vi "Begin_Tipper.vi"() -> (0 "error out":errorcluster)   [LabVIEW 2012]
uses:
  <vilib>/Rock Robotics/WPI/CAN/Jaguar/SubVIs/WPI_CANJaguar_BrakeCoastMode.ctl
  <vilib>/Rock Robotics/WPI/MotorControl/WPI_MotorControlOpenCANJaguar.vi
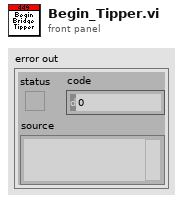
[diagram p1: front panel]
types:
  T1 = typedef "WPI_CANJaguar_BrakeCoastMode.ctl" = enum8{"Jumper", "Brake", "Coast"}
  T2 = typedef "WPI_MotorControlDeviceRef.ctl" = cluster{"DeviceStatus":errorcluster, "Type":enum16{"PWM", "CAN"}, "PWM":cluster{"Digital Module":T3, "PWM Channel":T4, "DeadBand":T5}, "CAN":cluster{"Device Number":u8, "Control Mode":T6, "Semaphore":T7, "Max Vout":dbl}, "Invert":bool, "TransformRef":T8, "InvTransformRef":T8}
  T3 = typedef "FPGA_TypedefDigitalModule.ctl" = enum16{"Digital Module 1", "Digital Module 2"}
  T4 = typedef "FPGA_DIOPWMChannel.ctl" = enum8{"PWM 1", "PWM 2", "PWM 3", "PWM 4", "PWM 5", "PWM 6", "PWM 7", "PWM 8", "PWM 9", "PWM 10", "Invalid"}
  T5 = typedef "WPI_PWMDeadband.ctl" = cluster{"Name":string, "maxPositivePwm":i32, "minPositivePwm":i32, "centerPwm":i32, "maxNegativePwm":i32, "minNegativePwm":i32, "angularRange":u16}
  T6 = typedef "WPI_CANJaguar_ControlMode.ctl" = enum8{"Percent VBus", "Current", "Speed", "Position", "Voltage"}
  T7 = typedef "Semaphore RefNum" = refnum<k1>
  T8 = typedef "WPI_PWMTransform_ConPane.ctl" = refnum<vi>
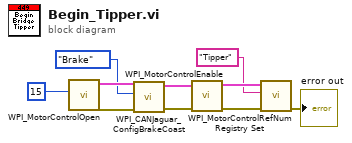
[diagram p0: block diagram]
diagram:
  n1 = call-poly <vilib>:"WPI_MotorControlOpen.vi"("Device Number"=u8 15) -> ("error out"=w3:errorcluster, "MotorControlDeviceRef"=w2:T2)  [unwired: 9 in]
  n2 = call <vilib>:"WPI_CANJaguar_ConfigBrakeCoast.vi"("error in (no error)"=w3, "Brake / Coast Mode"=WPI_CANJaguar_BrakeCoastMode."Brake", "CAN Jaguar Ref"=w2) -> ("error out"=w4:errorcluster, "CAN Jaguar Ref Out"=w5:T2)  [unwired: 7 in]
  n3 = call <vilib>:"WPI_MotorControlEnable.vi"("error in (no error)"=w4, "CAN Jaguar Ref"=w5) -> ("error out"=w9:errorcluster, "CAN Jaguar Ref Out"=w8:T2)  [unwired: 8 in]
  n4 = call <vilib>:"WPI_MotorControlRefNum Registry Set.vi"("error in (no error)"=w9, "refnum name"="Tipper", "MotorControlDevRef"=w8) -> ("error out"=→"error out":errorcluster)  [unwired: 7 in, 1 out]
